vi "N6701A_Initialize.vi"(8 "error in (no error)":errorcluster, 10 "Reset?":bool=TRUE, 11 "String":string="PS2") -> (0 "error out":errorcluster, 3 "VISA resource name out":refnum<visa-resource-name>)   [LabVIEW 2015]
uses:
  <instrlib>/Agilent N6700 Series/Agilent N6700 Series.lvlib
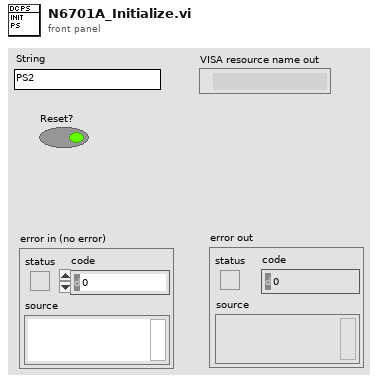
[diagram p1: front panel]
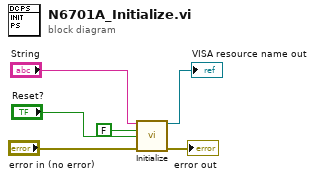
[diagram p0: block diagram]
diagram:
  n1 = call <instrlib>:"Initialize.vi"("VISA resource name"="String", "ID Query? (T: Yes)"=FALSE, "Reset? (T: Yes)"="Reset?", "error in (no error)"="error in (no error)") -> ("VISA resource name out"=→"VISA resource name out":refnum<visa-resource-name>, "error out"=→"error out":errorcluster)  [unwired: 10 in]
